vi "Camera Manager Get Camera Name.vi"(8 "error in (no error)":errorcluster, 11 "cameraId":i32) -> (0 "error out":errorcluster, 2 "Name out":string)   [LabVIEW 2017, in "PlayNitrideCameraComponet1010_4.lvlib"]
doc: "__declspec(dllexport) void CameraManager_GetCameraName(int cameraId, char* Name);"
uses:
  <userlib>/PlayNitrideCameraComponet1010_4/PlayNitrideCameraComponet1010_4.lvlib
  <userlib>/PlayNitrideCameraComponet1010_4/PlayNitrideCameraComponet.dll
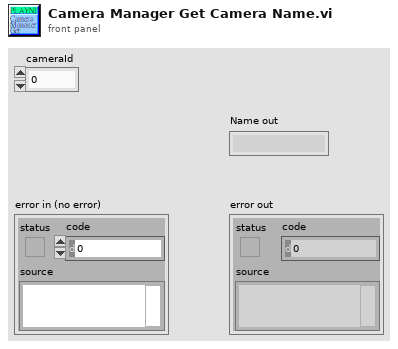
[diagram p1: front panel]
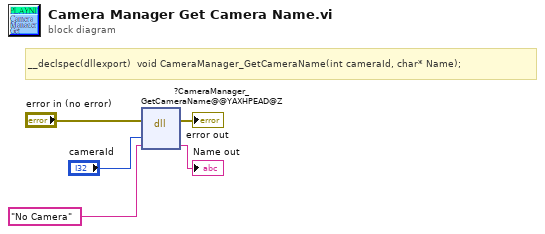
[diagram p0: block diagram]
diagram:
  # "__declspec(dllexport)  void CameraManager_GetCameraName(int cameraId, char* Name);"
  n1 = dll-call lib="C:/Program Files/National Instruments/LabVIEW 2017/user.lib/PlayNitrideCameraComponet1010_4/PlayNitrideCameraComponet.*" fn="?CameraManager_GetCameraName@@YAXHPEAD@Z"(error in="error in (no error)", "cameraId"="cameraId", "Name"="No Camera") -> (error out=→"error out":errorcluster, "Name"=→"Name out":string)  [unwired: 4 in, 1 out]
